vi "Configuration Complete_5160.vi"(8 "error in":errorcluster, 11 "FPGA VI Reference":T1) -> (0 "error out":errorcluster, 2 "Configured?":bool, 3 "FPGA VI Reference out":T1)   [LabVIEW 2013]
uses:
  5160FPGAref.ctl
  <vilib>/rvi/interface/common/niFpgaWaitOnOcc.vi
  <vilib>/Utility/error.llb/Error Cluster From Error Code.vi
  <vilib>/rvi/errors/niLvFpgaAdjustHostInterfaceError.vi
  <vilib>/rvi/interface/nirviReadWriteControl/nirviReadWriteControl.xnode
  NiFpgaLv.dll
  <vilib>/rvi/interface/Simulation/niFpgaSimulationCallBeginRW.vi
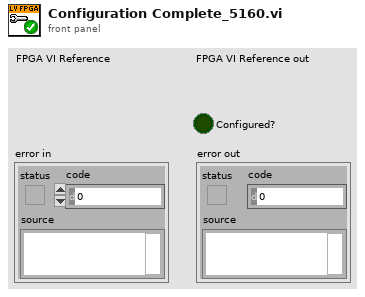
[diagram p1: front panel]
types:
  T1 = typedef "5160FPGAref.ctl" = refnum<k20>
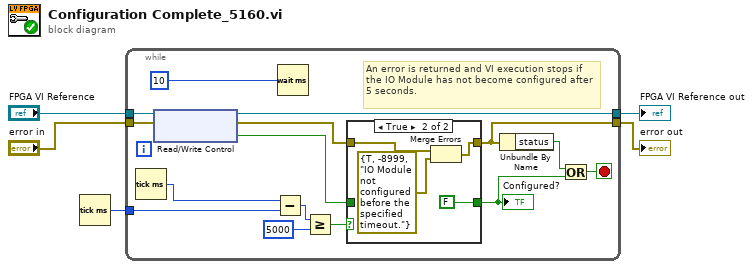
[diagram p0: block diagram]
diagram:
  n1 = Tick Count (ms)() -> (millisecond timer value=w1:u32)
  n2 = while {
    tunnel: "error in" -> [w13]
    tunnel: [w17] -> w4
    tunnel: [w9] -> w2
    tunnel: "FPGA VI Reference" -> [w12]
    tunnel: w1 -> [w7]
    stop <- w15 stop-if-true
    # "An error is returned and VI execution stops if the IO Module has not become configured after 5 seconds."
    n3 = Tick Count (ms)() -> (millisecond timer value=w8:u32)
    n4 = xnode "Read/Write Control"("FPGA VI Reference In"=w12, "error in"=w13) -> ("FPGA VI Reference Out"=w9:T1, "error out"=w10:errorcluster, "Configured?"=w11:bool)
    n5 = Subtract(x=w8, y=w7) -> (x-y=w6:u32)
    n6 = Wait (ms)(milliseconds to wait=u32 10) -> ()  [unwired: 1 out]
    n7 = Greater Or Equal?(x=w6, y=u32 5000) -> (x >= y?=w18:bool)
    n8 = case shown="True" w18 {
      tunnel: [w22 FALSE ("Configured?")] -> w14
      tunnel: w11 -> [w22 _]
      tunnel: [w21 w25] -> w17
      tunnel: w10 -> [w21 w23]
      frame False {
      }
      frame True {
        n9 = Merge Errors(w23, errorcluster {"status"=TRUE, "code"=-8999, "source"="IO Module not configured before the specified timeout."} ("error in")) -> (w25:errorcluster)
      }
    }
    "Configured?" <- w14
    n10 = Unbundle By Name(w17) -> ("status"=w16:bool)
    n11 = Or(x=w16, y=w14) -> (x .or. y?=w15:bool)
  }
  "error out" <- w4
  "FPGA VI Reference out" <- w2
